vi "S2DS_ComputeWC.vi"(8 "error in (no error)":errorcluster, 9 "Parsed Formula Node":T1 {"Y Values" format="%.2f"}, 10 "WC info in":T2) -> (0 "error out":errorcluster, 2 "WC info out":T2)   [LabVIEW 2025]
uses:
  TYPE DEFS/S2DS_WC info.ctl
  TYPE DEFS/S2DS_Single WC info.ctl
  <vilib>/gmath/NI_Gmath.lvlib
panel:
  # "operator"
  # "register1"
  # "register2"
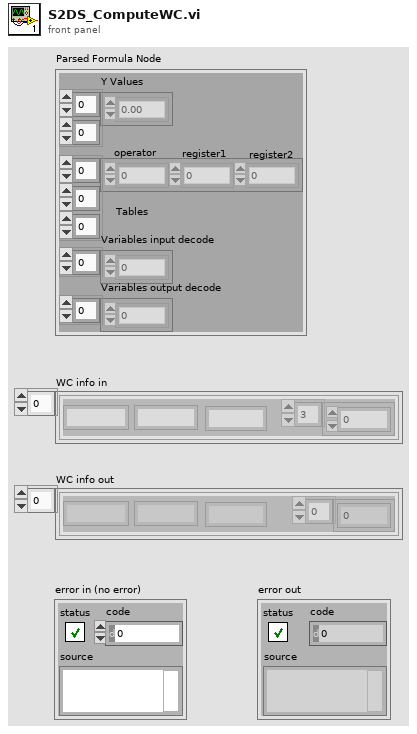
[diagram p1: front panel]
types:
  T1 = cluster{"Y Values":dbl[][], "Tables":i32[][][], "Variables input decode":i32[], "Variables output decode":i32[]}
  T2 = typedef "S2DS_WC info.ctl" = T3[]
  T3 = typedef "S2DS_Single WC info.ctl" = cluster{"Instrument identifier":string, "Write channel parameters":dbl[], "Name":string, "Unit":string}
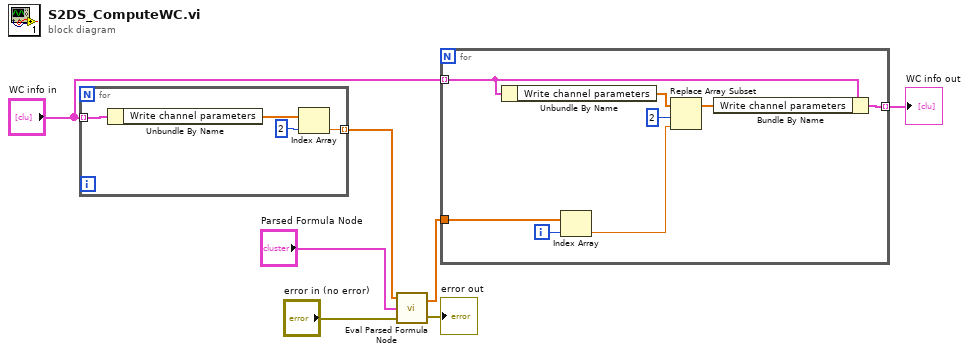
[diagram p0: block diagram]
diagram:
  n1 = for {
    tunnel: "WC info in" -> [w11] mode=indexing
    tunnel: [w8] -> w7 mode=indexing
    n2 = Unbundle By Name(w11) -> ("Write channel parameters"=w10:dbl[])
    n3 = Index Array(array=w10, index=2) -> (element=w8:dbl)
  }
  n4 = call <vilib>:"Eval Parsed Formula Node.vi"("error in (no error)"="error in (no error)", "Parsed Formula Node"="Parsed Formula Node", "Input Values"=w7) -> ("error out"=→"error out":errorcluster, "Output Values"=w6:dbl[])
  n5 = for {
    tunnel: w6 -> [w14]
    tunnel: "WC info in" -> [w17] mode=indexing
    tunnel: [w15] -> w1 mode=indexing
    i -> [w13]
    n6 = Unbundle By Name(w17) -> ("Write channel parameters"=w19:dbl[])
    n7 = Index Array(array=w14, index=w13) -> (element=w12:dbl)
    n8 = Replace Array Subset(array=w19, new element=w12, index=2) -> (w16:dbl[])
    n9 = Bundle By Name(cluster=w17, "Write channel parameters"=w16) -> (w15:T3)
  }
  "WC info out" <- w1
